vi "Create.vi"(8 "error in (no error)":errorcluster, 10 "Status":string) -> (0 "error out":errorcluster, 3 "Send-status out":refnum<class "Send-status.lvclass">)   [LabVIEW 2013, in "Messages.lvlib" / "Send-status.lvclass"]
uses:
  Send-status.lvclass
  Base-messages.ctl
  Send-status.lvclass/Send-status.ctl
  Messages.lvlib
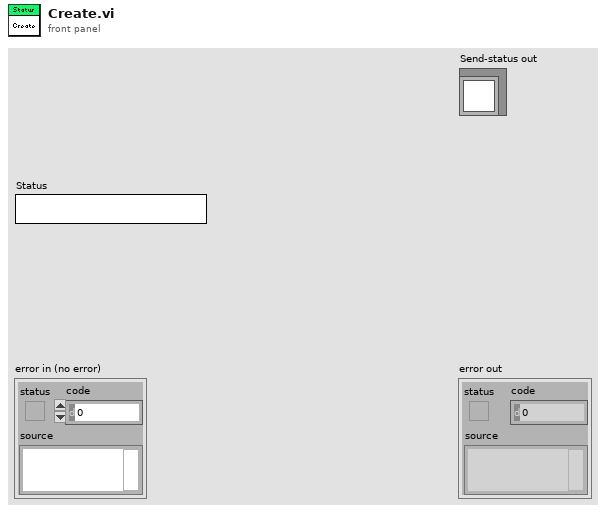
[diagram p1: front panel]
types:
  T1 = typedef "Messages.lvlib/Base-messages.ctl" = enum16{"Heartbeat", "Error", "Start client", "Stop client", "Get clients", "Query status", "Send status", "Action"}
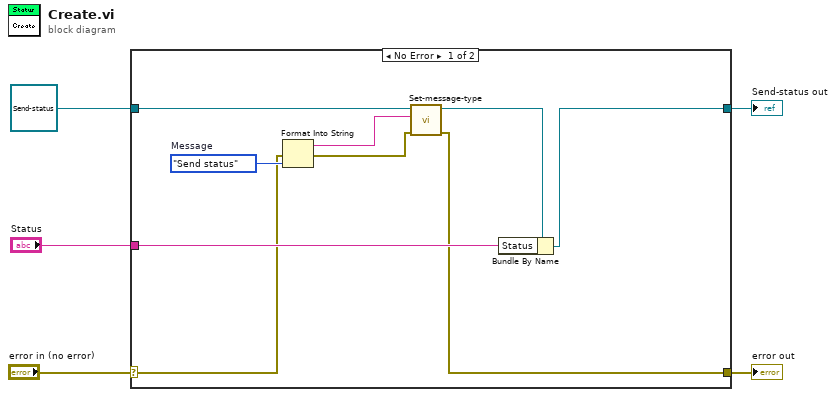
[diagram p0: block diagram]
diagram:
  n1 = case shown="No Error" "error in (no error)" {
    selector: "error in (no error)" -> [w7 w16]
    tunnel: [w10 w16] -> w4
    tunnel: [w12 w15] -> w2
    tunnel: refnum<class "Send-status.lvclass"> refnum ("Send-status") -> [w14 w15]
    tunnel: "Status" -> [w11 _]
    frame No Error {
      w9 = Base-messages."Send status"  # Message
      n2 = Format Into String(error in=w7, w9) -> (resulting string=w8:string, error out=w6:errorcluster)  [unwired: 2 in]
      n3 = call-dynamic "Set-message-type.vi"("error in (no error)"=w6, "Message type"=w8, "Message in"=w14) -> ("error out"=w10:errorcluster, "Message out"=w13:refnum<class "Send-status.lvclass">)  [unwired: 7 in]
      n4 = Bundle By Name(cluster=w13, "Status"=w11) -> (w12:refnum<class "Send-status.lvclass">)
    }
    frame Error {
    }
  }
  "error out" <- w4
  "Send-status out" <- w2
